vi "randco.vi"(1 "Array":string[](array[string])) -> (0 "appended array":string[](array[string]))   [LabVIEW 2019]
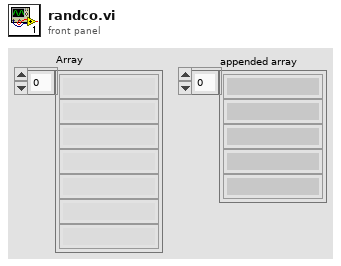
[diagram p1: front panel]
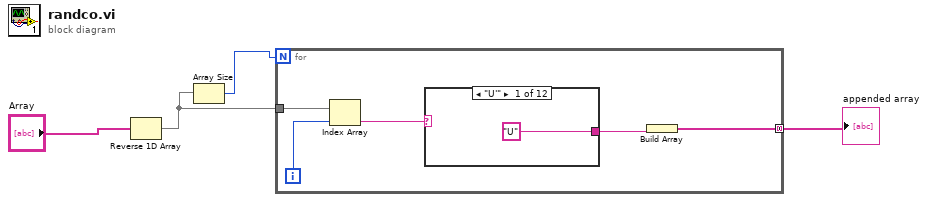
[diagram p0: block diagram]
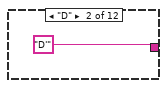
[diagram p2: hidden frame]
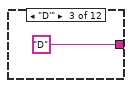
[diagram p3: hidden frame]
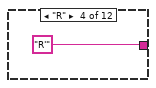
[diagram p4: hidden frame]
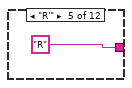
[diagram p5: hidden frame]
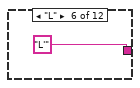
[diagram p6: hidden frame]
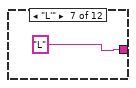
[diagram p7: hidden frame]
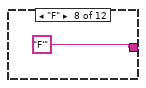
[diagram p8: hidden frame]
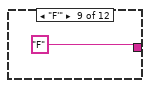
[diagram p9: hidden frame]
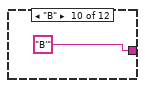
[diagram p10: hidden frame]
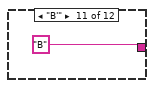
[diagram p11: hidden frame]
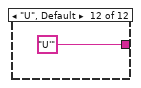
[diagram p12: hidden frame]
diagram:
  n1 = Reverse 1D Array(array="Array") -> (reversed array=w2:string[])
  n2 = Array Size(array=w2) -> (size(s)=w3:i32)
  n3 = for {
    N: w3 -> [_]
    tunnel: w2 -> [w8]
    tunnel: [w5] -> w1 mode=concatenating
    i -> [w9]
    n4 = Index Array(array=w8, index=w9) -> (element=w7:string)
    n5 = case shown="\"U'\"" w7 {
      tunnel: ["U" "D'" "D" "R'" "R" "L'" "L" "F'" "F" "B'" "B" "U'"] -> w6
      frame "U'" {
      }
      frame "D" {
      }
      frame "D'" {
      }
      frame "R" {
      }
      frame "R'" {
      }
      frame "L" {
      }
      frame "L'" {
      }
      frame "F" {
      }
      frame "F'" {
      }
      frame "B" {
      }
      frame "B'" {
      }
      frame "U", Default {
      }
    }
    n6 = Build Array(w6) -> (w5:string[])
  }
  "appended array" <- w1
